vi "dpu_id_read.vi"(8 "error in":errorcluster, 11 "master":refnum<class "Modbus Master.lvclass">) -> (0 "error out":errorcluster, 2 "DPU_ID":T1={"HW_REV"=256, "FW_REV"=256, "NODE_SN"=256, "NODE_ADDR"=256, "NODE_TYPE"="product-name", "NODE_NAME"="node-name", "NODE_VEND"="", "RANGE_SEL"=0} {"RANGE_SEL" format="%0d"; "HW_REV" format="%04x"; "FW_REV" format="%04x"; "NODE_ADDR" format="%x"}, 3 "master out":refnum<class "Modbus Master.lvclass">)   [LabVIEW 2014]
uses:
  protocol/modbus/ni_modbus_api/API/Master/Modbus Master.lvclass
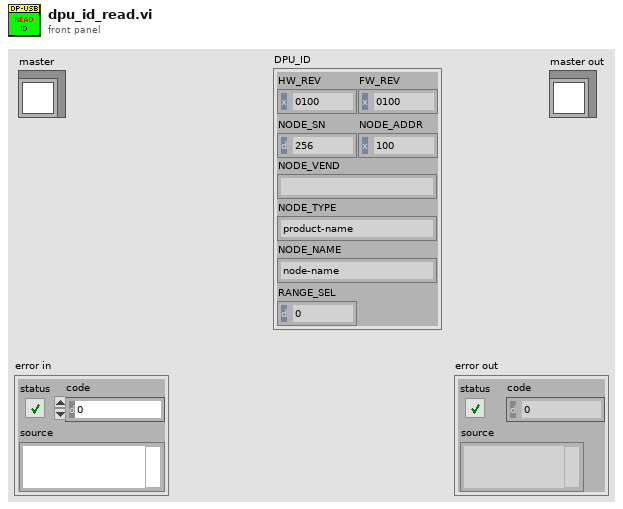
[diagram p1: front panel]
types:
  T1 = cluster{"HW_REV":u16, "FW_REV":u16, "NODE_SN":u32, "NODE_ADDR":u16, "NODE_TYPE":string, "NODE_NAME":string, "NODE_VEND":string, "RANGE_SEL":u16}
  T2 = enum16{"big-endian, network order", "native, host order", "little-endian"}
  T3 = cluster{"HW_REV":u16, "FW_REV":u16, "NODE_SN":u32, "NODE_ADDR":u16}
  T4 = cluster{"strings[0]":string, "strings[1]":string, "strings[2]":string}
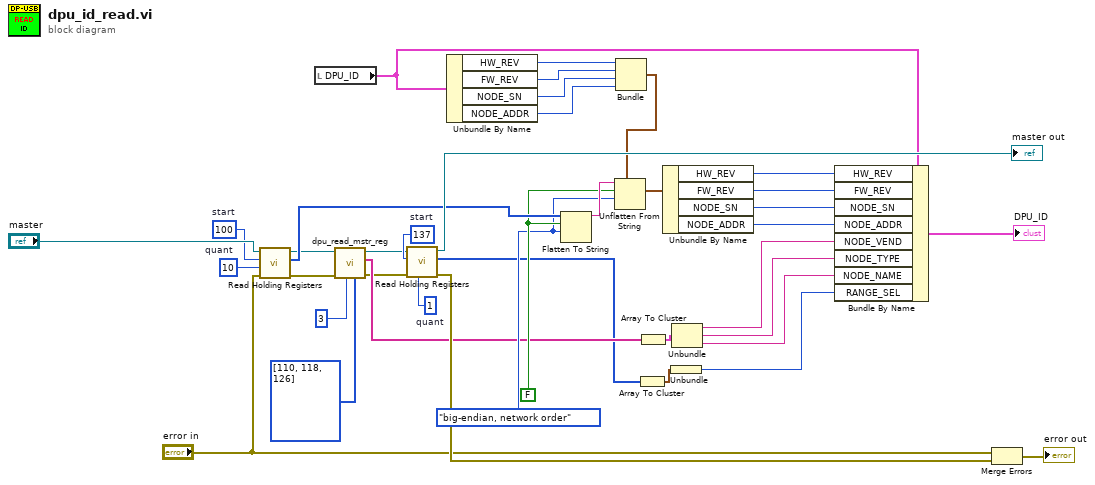
[diagram p0: block diagram]
diagram:
  w7 = u16 1  # quant
  w6 = u16 137  # start
  w17 = T2."big-endian, network order" ("byte order (0:big-endian, network order)")
  w18 = FALSE ("prepend array or string size? (T)")
  w31 = u16 10  # quant
  w32 = u16 100  # start
  n1 = call-dynamic "Read Holding Registers.vi"("error in"="error in", "number of inputs"=w31, "starting address"=w32, "Modbus master in"="master") -> ("error out"=w16:errorcluster, "register values"=w20:u16[], "Modbus master out"=w15:refnum<class "Modbus Master.lvclass">)  [unwired: 5 in]
  n2 = local read "DPU_ID"() -> (w19:T1)
  n3 = call "dpu_read_mstr_reg.vi"("str non-consec regs"=u16[] [110, 118, 126], "num of str"=u16 3, "error in"=w16, "master"=w15) -> ("error out"=w5:errorcluster, "strings"=w12:string[], "master out"=w4:refnum<class "Modbus Master.lvclass">)  [unwired: 4 in, 1 out]
  n4 = call-dynamic "Read Holding Registers.vi"("error in"=w5, "number of inputs"=w7, "starting address"=w6, "Modbus master in"=w4) -> ("error out"=w36:errorcluster, "register values"=w2:u16[], "Modbus master out"=→"master out":refnum<class "Modbus Master.lvclass">)  [unwired: 5 in]
  n5 = Unbundle By Name(w19) -> ("HW_REV"=w30:u16, "FW_REV"=w29:u16, "NODE_SN"=w28:u32, "NODE_ADDR"=w27:u16)
  n6 = Flatten To String(anything=w20, prepend array or string size? (T)=w18, byte order (0:big-endian, network order)=w17) -> (data string=w33:string)  [unwired: 1 in, 2 out]
  n7 = Bundle("HW_REV"=w30, "FW_REV"=w29, "NODE_SN"=w28, "NODE_ADDR"=w27) -> (w26:T3)  [unwired: 1 in]
  n8 = Unflatten From String(type=w26, binary string=w33, data includes array or string size? (T)=w18, byte order (0:big-endian, network order)=w17) -> (value=w25:T3)  [unwired: 1 in, 2 out]
  n9 = Array To Cluster(array=w2) -> (cluster=w3:cluster{"register values[0]":u16})
  n10 = Array To Cluster(array=w12) -> (cluster=w11:T4)
  n11 = Unbundle By Name(w25) -> ("HW_REV"=w24:u16, "FW_REV"=w23:u16, "NODE_SN"=w22:u32, "NODE_ADDR"=w21:u16)
  n12 = Unbundle(w3) -> ("register values[0]"=w1:u16)
  n13 = Unbundle(w11) -> ("strings[0]"=w10:string, "strings[1]"=w9:string, "strings[2]"=w8:string)
  n14 = Bundle By Name(cluster=w19, "HW_REV"=w24, "FW_REV"=w23, "NODE_SN"=w22, "NODE_ADDR"=w21, "NODE_VEND"=w10, "NODE_TYPE"=w9, "NODE_NAME"=w8, "RANGE_SEL"=w1) -> (→"DPU_ID":T1)
  n15 = Merge Errors("error in", w36) -> (→"error out":errorcluster)
